vi "test Log File.vi"(8 "error in":errorcluster, 11 "TestCase in":refnum<class "Embedded Data Logger Windows System Tests.lvclass">) -> (0 "error out":errorcluster, 3 "TestCase out":refnum<class "Embedded Data Logger Windows System Tests.lvclass">)   [LabVIEW 2027, in "Embedded Data Logger Windows System Tests.lvclass"]
uses:
  Embedded Data Logger Windows System Tests.lvclass
  65b597e9-841e-47e7-abef-1fad86639178.vi
  80b35fc5-226e-4f52-a2ba-c14ddf55d3b0.vi
  C:/Program Files/National Instruments/LabVIEW 2027/vi.lib/addons/_JKI Toolkits/VI Tester/TestCase.llb/TestCase.lvclass
  <vilib>/addons/_JKI Toolkits/VI Tester/TestCase.llb/TestCase.lvclass
panel:
  out "End Time":dbl
  out "Start Time":dbl
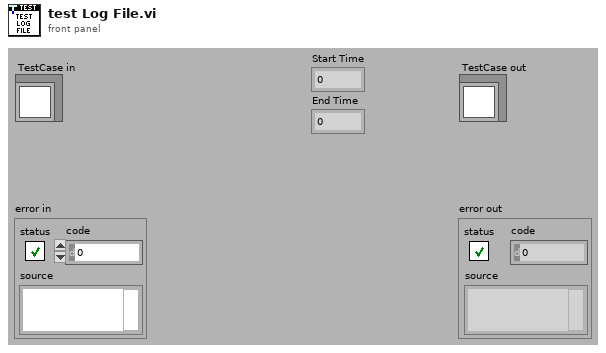
[diagram p1: front panel]
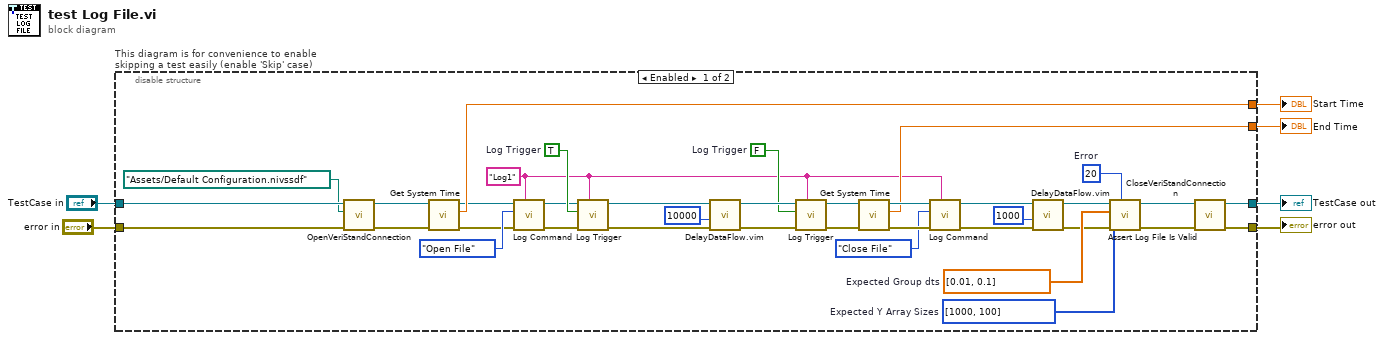
[diagram p0: block diagram]
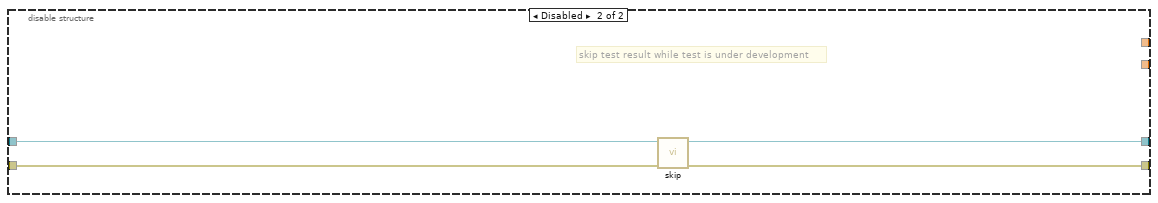
[diagram p2: hidden frame]
diagram:
  n1 = disable-structure "This diagram is for convenience to enable skipping a test easily (enable 'Skip' case)" shown="Enabled" {
    disable-tunnel: "TestCase in" -> [w26 w45]
    disable-tunnel: [w22 w43] -> w3
    disable-tunnel: [w23 w44] -> w5
    disable-tunnel: "error in" -> [w28 w42]
    disable-tunnel: [w31 _] -> w2
    disable-tunnel: [w30 _] -> w1
    frame Enabled {
      w19 = i32[] [1000, 100]  # Expected Y Array Sizes
      w20 = dbl[] [0.01, 0.1]  # Expected Group dts
      w13 = "Log1" ("Embedded Data Logger File Name")
      w32 = 20  # Error
      w38 = FALSE  # Log Trigger
      w40 = TRUE  # Log Trigger
      n2 = call-dynamic "OpenVeriStandConnection.vi"("error in (no error)"=w28, "System Definition File"=path "Assets/Default Configuration.nivssdf", "VeriStand Test Case in"=w26) -> ("error out"=w29:errorcluster, "VeriStand Test Case out"=w27:refnum<class "Embedded Data Logger Windows System Tests.lvclass">)  [unwired: 6 in, 1 out]
      n3 = call "Get System Time.vi"("error in (no error)"=w29, "Embedded Data Logger System Tests in"=w27) -> ("error out"=w17:errorcluster, "System Time"=w30:dbl, "Embedded Data Logger System Tests out"=w15:refnum<class "Embedded Data Logger Windows System Tests.lvclass">)  [unwired: 7 in]
      n4 = call "Log Command.vi"("Embedded Data Logger File Name"=w13, "error in"=w17, "Log Command"=enum16{"Idle", "Open File", "Close File"}."Open File", "Embedded Data Logger System Tests in"=w15) -> ("error out"=w16:errorcluster, "Embedded Data Logger System Tests out"=w14:refnum<class "Embedded Data Logger Windows System Tests.lvclass">)  [unwired: 6 in]
      n5 = call "Log Trigger.vi"("Embedded Data Logger File Name"=w13, "error in"=w16, "Log Trigger"=w40, "Embedded Data Logger System Tests in"=w14) -> ("error out"=w11:errorcluster, "Embedded Data Logger System Tests out"=w41:refnum<class "Embedded Data Logger Windows System Tests.lvclass">)  [unwired: 6 in]
      n6 = call "DelayDataFlow.vim"("value in"=w11, "milliseconds to wait"=u32 10000) -> ("value out"=w10:errorcluster)  [unwired: 2 in, 1 out]
      n7 = call "Log Trigger.vi"("Embedded Data Logger File Name"=w13, "error in"=w10, "Log Trigger"=w38, "Embedded Data Logger System Tests in"=w41) -> ("error out"=w36:errorcluster, "Embedded Data Logger System Tests out"=w39:refnum<class "Embedded Data Logger Windows System Tests.lvclass">)  [unwired: 6 in]
      n8 = call "Get System Time.vi"("error in (no error)"=w36, "Embedded Data Logger System Tests in"=w39) -> ("error out"=w34:errorcluster, "System Time"=w31:dbl, "Embedded Data Logger System Tests out"=w37:refnum<class "Embedded Data Logger Windows System Tests.lvclass">)  [unwired: 7 in]
      n9 = call "Log Command.vi"("Embedded Data Logger File Name"=w13, "error in"=w34, "Log Command"=enum16{"Idle", "Open File", "Close File"}."Close File", "Embedded Data Logger System Tests in"=w37) -> ("error out"=w8:errorcluster, "Embedded Data Logger System Tests out"=w35:refnum<class "Embedded Data Logger Windows System Tests.lvclass">)  [unwired: 6 in]
      n10 = call "DelayDataFlow.vim"("value in"=w8, "milliseconds to wait"=u32 1000) -> ("value out"=w7:errorcluster)  [unwired: 2 in, 1 out]
      n11 = call "Assert Log File Is Valid.vi"("Error"=w32, "error in"=w7, "Expected Y Array Sizes"=w19, "Expected Group dts"=w20, "Embedded Data Logger System Tests in"=w35) -> ("error out"=w24:errorcluster, "Embedded Data Logger System Tests out"=w21:refnum<class "Embedded Data Logger Windows System Tests.lvclass">)  [unwired: 5 in]
      n12 = call-dynamic "CloseVeriStandConnection.vi"("error in (no error)"=w24, "VeriStand Test Case in"=w21) -> ("error out"=w23:errorcluster, "VeriStand Test Case out"=w22:refnum<class "Embedded Data Logger Windows System Tests.lvclass">)  [unwired: 8 in]
    }
    frame Disabled {
      # "skip test result while test is under development"
      n13 = call <vilib>:"skip.vi"("error in (no error)"=w42, "TestCase in"=w45) -> ("error out"=w44:errorcluster, "TestCase out"=w43:refnum<class "Embedded Data Logger Windows System Tests.lvclass">)  [unwired: 8 in]
    }
  }
  "error out" <- w5
  "TestCase out" <- w3
  "Start Time" <- w1
  "End Time" <- w2
